vi "load.vi"(8 "error in (no error)":errorcluster) -> (0 "error out":errorcluster)   [LabVIEW 2016, in "环境动力监测库.lvlib"]
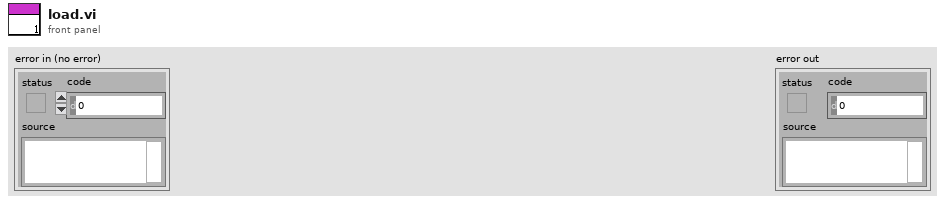
[diagram p1: front panel]
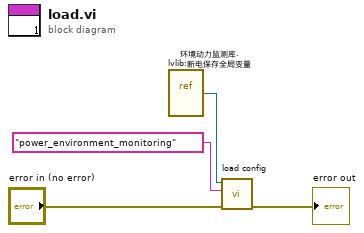
[diagram p0: block diagram]
diagram:
  n1 = vi-ref "环境动力监测库.lvlib:断电保存全局变量.vi"() -> (w3:refnum<vi>)
  n2 = call "load config.vi"("error in (no error)"="error in (no error)", "TABLE"="power_environment_monitoring", "VI引用句柄"=w3) -> ("error out"=→"error out":errorcluster)  [unwired: 8 in]
